vi "Copy.vi"(0 "Conditional in":refnum<class "Conditional.lvclass">, 1 "Linked List Ref":refnum<data-value>, 2 "New Parent ID":string, 5 "Test ID":string, 7 "Insertion Index":i32=-1, 9 "Move?":bool, 11 "error in (no error)":errorcluster, 12 "New ID":string, 13 "Data IDs":variant) -> (3 "Linked List Ref out":refnum<data-value>, 6 "Linked List ID out":string, 14 "Data IDs out":variant, 15 "error out":errorcluster)   [LabVIEW 2017, in "Test Executive.lvlib" / "Conditional.lvclass"]
uses:
  <vilib>/gpm_packages/@cs/test-executive/Source/Test Executive/Conditional/Conditional.lvclass
  <vilib>/gpm_packages/@cs/linked-list/Source/Linked List/ILinkedList/ILinked List.lvclass
  <vilib>/gpm_packages/@cs/test-executive/Source/Test Executive/Executioner/Executioner.lvclass
  170d0bf8-3ce4-4b61-beee-8de6a9555dcd.vi
  8c6f9ea9-cb7b-4d30-8c6c-37deb1dc3811.vi
  439bdb0e-a58c-4a1e-b65e-cefac105e484.vi
  28a4d2c3-02d8-45de-ad56-a7f6d6817309.vi
  <vilib>/gpm_packages/@cs/linked-list/Source/Linked List/Linked List Ref/Linked List Ref.lvclass
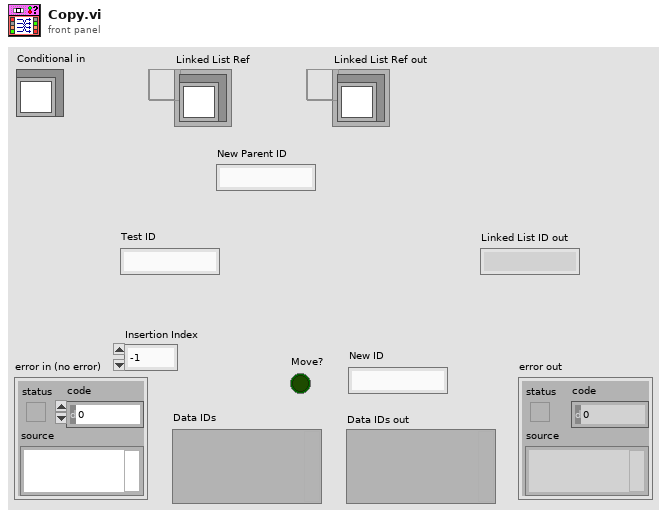
[diagram p1: front panel]
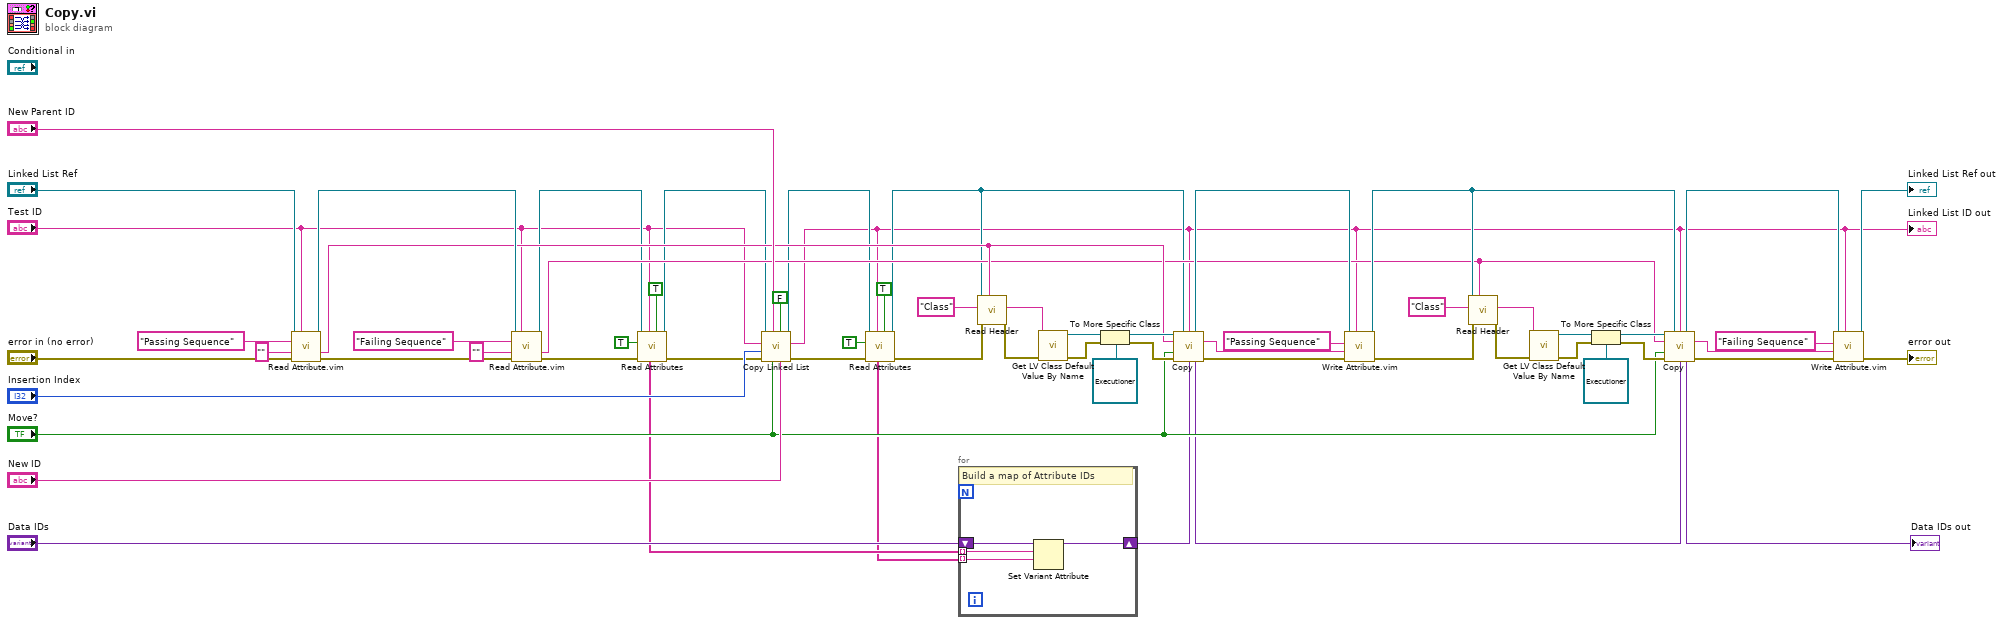
[diagram p0: block diagram]
diagram:
  n1 = call "Read Attribute.vim"("Linked List Ref"="Linked List Ref", "Linked List ID"="Test ID", "Attribute Name"="Passing Sequence", "Type"="", "error in (no error)"="error in (no error)") -> ("Linked List Ref out"=w52:refnum<data-value>, "Attribute"=w22:string, "error out"=w53:errorcluster)  [unwired: 5 in, 3 out]
  n2 = call "Read Attribute.vim"("Linked List Ref"=w52, "Linked List ID"="Test ID", "Attribute Name"="Failing Sequence", "Type"="", "error in (no error)"=w53) -> ("Linked List Ref out"=w7:refnum<data-value>, "Attribute"=w21:string, "error out"=w9:errorcluster)  [unwired: 5 in, 3 out]
  n3 = call <vilib>:"Read Attributes.vi"("Flatten Pointer?"=TRUE, "Linked List ID"="Test ID", "error in (no error)"=w9, "Include Private?"=TRUE, "Linked List Ref"=w7) -> ("error out"=w8:errorcluster, "Linked List Ref out"=w6:refnum<data-value>, "Data IDs"=w2:string[])  [unwired: 1 in, 3 out]
  n4 = call <vilib>:"Copy Linked List.vi"("New Linked List ID"="New ID", "Recursive? (T)"=FALSE, "Move?"="Move?", "New Parent Linked List ID"="New Parent ID", "error in (no error)"=w8, "Insertion Index"="Insertion Index", "Linked List ID"="Test ID", "Linked List Ref"=w6) -> ("error out"=w18:errorcluster, "Linked List ID out"=w14:string, "Linked List Ref out"=w16:refnum<data-value>)  [unwired: 1 out]
  "Linked List ID out" <- w14
  n5 = call <vilib>:"Read Attributes.vi"("Flatten Pointer?"=TRUE, "Linked List ID"=w14, "error in (no error)"=w18, "Include Private?"=TRUE, "Linked List Ref"=w16) -> ("error out"=w17:errorcluster, "Linked List Ref out"=w15:refnum<data-value>, "Data IDs"=w1:string[])  [unwired: 1 in, 3 out]
  n6 = for {
    tunnel: w2 -> [w66] mode=indexing
    tunnel: w1 -> [w65] mode=indexing
    shift-right: [w64] -> w3
    shift-left: "Data IDs" -> [w67]
    # "Build a map of Attribute IDs"
    n7 = Set Variant Attribute(Variant=w67, name=w66, value=w65) -> (Variant out=w64:variant)  [unwired: 1 in, 2 out]
  }
  n8 = call <vilib>:"Read Header.vi"("Linked List ID"=w22, "error in (no error)"=w17, "Header Name"="Class", "Linked List Ref"=w15) -> ("error out"=w48:errorcluster, "Header Value"=w50:string)  [unwired: 4 in, 2 out]
  n9 = call <vilib>:"Get LV Class Default Value By Name.vi"("error in (no error)"=w48, "class name"=w50) -> ("error out"=w47:errorcluster, "object"=w49:refnum<class>)  [unwired: 8 in]
  n10 = To More Specific Class(target class=refnum<class "Executioner.lvclass"> refnum ("Test Executive.lvlib:Executioner.lvclass"), reference=w49, error in=w47) -> (specific class reference=w44:refnum<class "Executioner.lvclass">, error out=w45:errorcluster)
  n11 = call-dynamic "Copy.vi"("Executioner in"=w44, "Linked List Ref"=w15, "New Parent ID"=w14, "Test ID"=w22, "Move?"="Move?", "error in (no error)"=w45, "Data IDs"=w3) -> ("Linked List Ref out"=w40:refnum<data-value>, "Linked List ID out"=w41:string, "Data IDs out"=w13:variant, "error out"=w43:errorcluster)  [unwired: 5 in]
  n12 = call "Write Attribute.vim"("Linked List ID"=w14, "error in (no error)"=w43, "Attribute"=w41, "Attribute Name"="Passing Sequence", "Linked List Ref"=w40) -> ("error out"=w26:errorcluster, "Linked List Ref out"=w27:refnum<data-value>)  [unwired: 3 in, 2 out]
  n13 = call <vilib>:"Read Header.vi"("Linked List ID"=w21, "error in (no error)"=w26, "Header Name"="Class", "Linked List Ref"=w27) -> ("error out"=w31:errorcluster, "Header Value"=w29:string)  [unwired: 4 in, 2 out]
  n14 = call <vilib>:"Get LV Class Default Value By Name.vi"("error in (no error)"=w31, "class name"=w29) -> ("error out"=w32:errorcluster, "object"=w30:refnum<class>)  [unwired: 8 in]
  n15 = To More Specific Class(target class=refnum<class "Executioner.lvclass"> refnum ("Test Executive.lvlib:Executioner.lvclass"), reference=w30, error in=w32) -> (specific class reference=w35:refnum<class "Executioner.lvclass">, error out=w34:errorcluster)
  n16 = call-dynamic "Copy.vi"("Executioner in"=w35, "Linked List Ref"=w27, "New Parent ID"=w14, "Test ID"=w21, "Move?"="Move?", "error in (no error)"=w34, "Data IDs"=w13) -> ("Linked List Ref out"=w39:refnum<data-value>, "Linked List ID out"=w38:string, "Data IDs out"=→"Data IDs out":variant, "error out"=w36:errorcluster)  [unwired: 5 in]
  n17 = call "Write Attribute.vim"("Linked List ID"=w14, "error in (no error)"=w36, "Attribute"=w38, "Attribute Name"="Failing Sequence", "Linked List Ref"=w39) -> ("error out"=→"error out":errorcluster, "Linked List Ref out"=→"Linked List Ref out":refnum<data-value>)  [unwired: 3 in, 2 out]
